vi "From JSON.vi"(8 "error in (no error)":errorcluster, 11 "JSON":string) -> (0 "error out":errorcluster, 3 "Developer Group out":refnum<class "Developer Group.lvclass">)   [LabVIEW 2020, in "GCentral-API.lvlib" / "Developer Group.lvclass"]
uses:
  Developer Group.lvclass
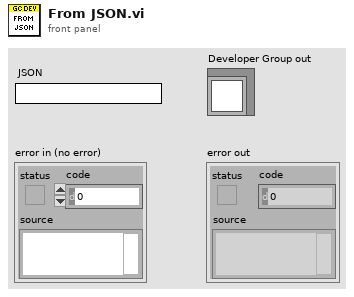
[diagram p1: front panel]
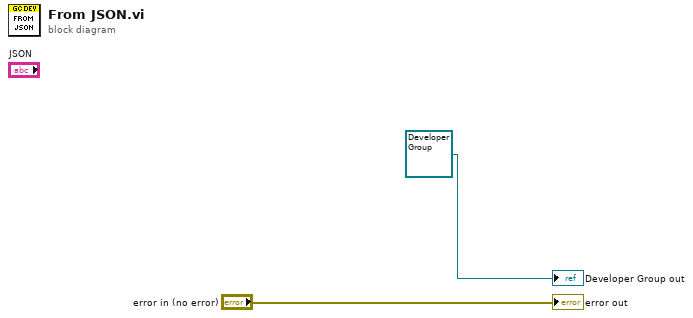
[diagram p0: block diagram]
diagram:
  "error out" <- "error in (no error)"
  "Developer Group out" <- refnum<class "Developer Group.lvclass"> refnum ("Developer Group in")
